vi "ConnectIVIsampleswitch.vi"(2 "error in (no error)":errorcluster, 3 "channel 2 (\"\")":string, 4 "channel 1 (\"\")":string, 5 "instrument handle in":refnum<k15>) -> (0 "error out":errorcluster, 1 "instrument handle out":refnum<k15>)   [LabVIEW 2012]
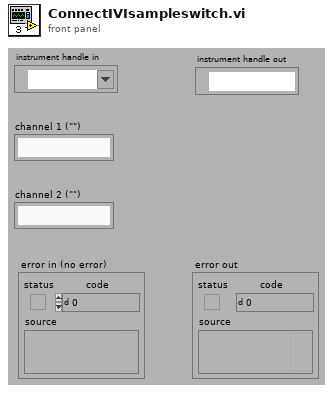
[diagram p1: front panel]
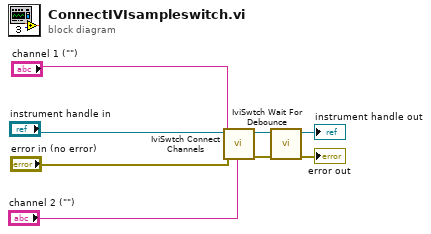
[diagram p0: block diagram]
diagram:
  n1 = call <vilib>:"IviSwtch Connect Channels.vi"("error in (no error)"="error in (no error)", "channel 2 (\"\")"="channel 2 (\"\")", "channel 1 (\"\")"="channel 1 (\"\")", "instrument handle"="instrument handle in") -> ("error out"=w4:errorcluster, "instrument handle out"=w3:refnum<k15>)  [unwired: 6 out]
  n2 = call <vilib>:"IviSwtch Wait For Debounce.vi"("error in (no error)"=w4, "instrument handle"=w3) -> ("error out"=→"error out":errorcluster, "instrument handle out"=→"instrument handle out":refnum<k15>)  [unwired: 1 in, 7 out]
